vi "RoomWithBombParamsStack.vi"(8 "error in (no error)":errorcluster, 10 "Bomb":bool, 11 "RoomNumber":i32) -> (0 "error out":errorcluster, 2 "HierarchyParams":variant[](array[variant]), 3 "RoomWithBomb":refnum<class "RoomWithBomb.lvclass">)   [LabVIEW 2020, in "RoomWithBomb.lvclass"]
uses:
  RoomWithBomb.lvclass
  E:/GitHub/Design-Patterns-GoF_-_NI-LV/Creational/GoFcommonClasses/ConcreteMazeSite/Room/Room.lvclass
  Room/Protected/property/Read RoomParams.vi
  Protected/property/Read BombedWallParams.vi
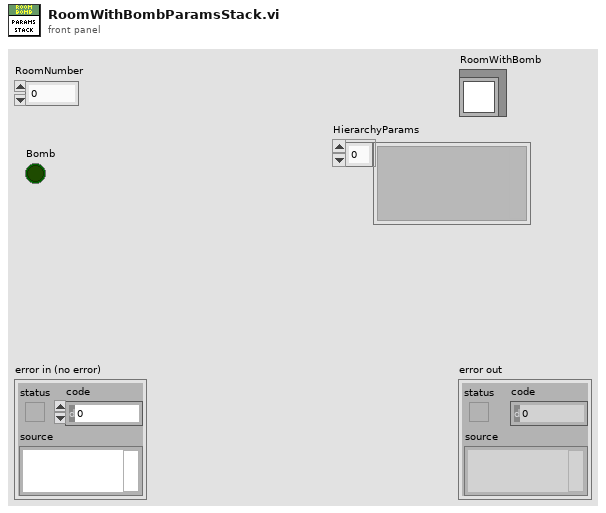
[diagram p1: front panel]
types:
  T1 = typedef "Room.lvclass/RoomParams.ctl" = cluster{"roomNumber":i32}
  T2 = typedef "RoomWithBomb.lvclass/RoomWithBombParams.ctl" = cluster{"bomb":bool}
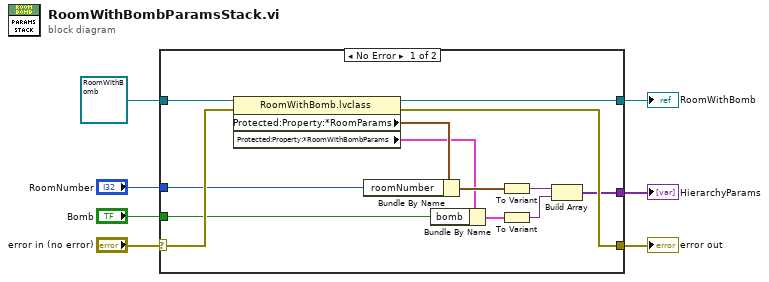
[diagram p0: block diagram]
diagram:
  n1 = case shown="No Error" "error in (no error)" {
    selector: "error in (no error)" -> [w20 w22]
    tunnel: [w17 w22] -> w6
    tunnel: "Bomb" -> [w12 _]
    tunnel: refnum<class "RoomWithBomb.lvclass"> refnum ("Milk") -> [w19 w21]
    tunnel: [w18 w21] -> w4
    tunnel: [w16 _] -> w3
    tunnel: "RoomNumber" -> [w10 _]
    frame No Error {
      n2 = property class="RoomWithBomb.lvclass"(reference=w19, error in=w20) -> (reference out=w18:refnum<class "RoomWithBomb.lvclass">, error out=w17:errorcluster, "Protected:Property:*RoomParams"=w13:T1, "Protected:Property:*RoomWithBombParams"=w11:T2)
      n3 = Bundle By Name(cluster=w13, "roomNumber"=w10) -> (w15:T1)
      n4 = Bundle By Name(cluster=w11, "bomb"=w12) -> (w8:T2)
      n5 = To Variant(anything=w15) -> (Variant=w14:variant)
      n6 = To Variant(anything=w8) -> (Variant=w9:variant)
      n7 = Build Array(w14, w9) -> (w16:variant[])
    }
    frame Error {
    }
  }
  "error out" <- w6
  "RoomWithBomb" <- w4
  "HierarchyParams" <- w3
